vi "datalogging_sub.vi"(8 "Center Goal Position":i8, 9 "Path Selected":string, 10 "States Executed":T2[](array[typedef]), 11 "NXT/EV3 In":T1) -> (3 "NXT/EV3 Out":T1)   [LabVIEW 2012, in "Mecanum Drive.lvrbt"]
uses:
  Mecanum Drive.lvrbt
  State_Typ.ctl
  <vilib>/NXT/Subs/LVHSConnector.ctl
  <vilib>/NXT/LegoClasses/BrickReference/BrickReference.lvclass
  <vilib>/NXT/NXTIO Xnodes/NXTIONodeSubVIs/LEGOStopAllMotors.vi
  <vilib>/NXT/NXTIO Xnodes/NXTIONodeSubVIs/LEGOMoveAllMotors.vi
  <vilib>/NXT/NXTIO Xnodes/NXTIOXNode/NXTIO.xnode
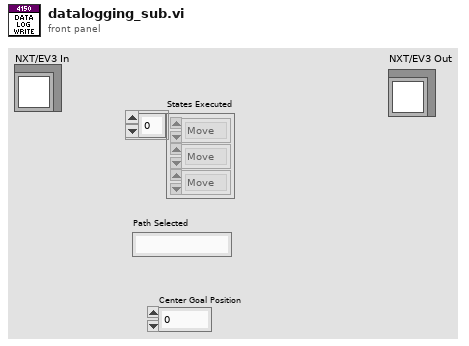
[diagram p1: front panel]
types:
  T1 = typedef "LVHSConnector.ctl" = refnum<class "BrickReference.lvclass">
  T2 = typedef "State_Typ.ctl" = enum16{"Move", "Check for Position 2", "Check for Position 3", "Stop"}
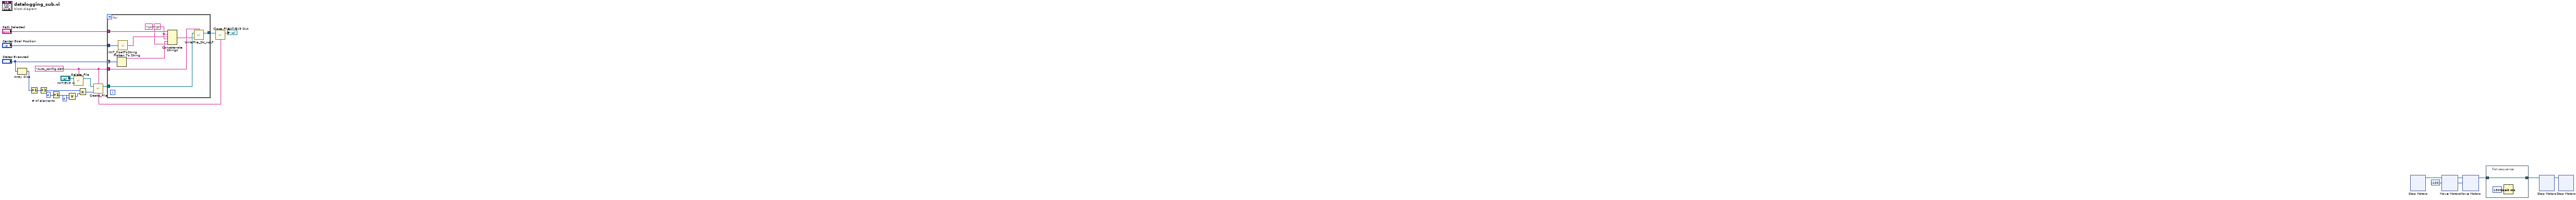
[diagram p0: block diagram]
diagram:
  w13 = 4  # # of elements
  w3 = "Auto_config.dat" ("Filename")
  w21 = i8 -100 ("Power/Speed 1")
  n1 = Array Size(array="States Executed") -> (size(s)=w6:i32)
  n2 = Increment(x=w6) -> (x+1=w14:i32)
  n3 = Increment(x=w14) -> (x+1=w9:i32)
  n4 = Increment(x=w13) -> (x+1=w12:i32)
  n5 = Multiply(x=w12, y=u32 4) -> (x*y=w11:u32)
  n6 = call <vilib>:"Delete_File.vi"("NXT/EV3"="NXT/EV3 In", "Filename"=w3) -> ("NXT/EV3"=w8:T1)  [unwired: 2 in]
  n7 = Multiply(x=w9, y=w11) -> (x*y=w15:u32)
  n8 = call <vilib>:"Create_File.vi"("File Size (256)"=w15, "NXT/EV3"=w8, "Filename"=w3) -> ("NXT/EV3"=w5:T1)  [unwired: 1 out]
  n9 = for {
    tunnel: "Path Selected" -> [w31]
    tunnel: "Center Goal Position" -> [w32]
    tunnel: "States Executed" -> [w26] mode=indexing
    tunnel: w5 -> [w34]
    tunnel: w3 -> [w24]
    tunnel: [w33] -> w4
    w29 = "\\t" ("string")
    n10 = Flatten To String(anything=w26) -> (data string=w25:string)  [unwired: 3 in, 2 out]
    n11 = call <vilib>:"NXT_floatToString.vi"("number"=w32) -> ("string"=w28:string)
    n12 = Concatenate Strings(w31, w29, w28, w29, w25, "\\n" ("string")) -> (w30:string)
    n13 = call <vilib>:"WriteFile_Str_noLF.vi"("String"=w30, "NXT/EV3"=w34, "Filename"=w24) -> ("NXT/EV3"=w33:T1)  [unwired: 1 in]
  }
  n14 = call <vilib>:"Close_File.vi"("NXT/EV3"=w4, "Filename"=w3) -> ("NXT/EV3"=→"NXT/EV3 Out":T1)  [unwired: 2 in]
  n15 = xnode "Stop Motors"() -> ("NXT/EV3"=w16:T1)  [unwired: 2 in]
  n16 = xnode "Move Motors"("Power/Speed 1"=w21, "NXT/EV3"=w16) -> ("NXT/EV3"=w20:T1)  [unwired: 1 in]
  n17 = xnode "Move Motors"("Power/Speed 1"=w21, "NXT/EV3"=w20) -> ("NXT/EV3"=w17:T1)  [unwired: 1 in]
  n18 = flat-sequence {
    tunnel: [w35] -> w19
    tunnel: w17 -> [w35]
    frame #0 {
      n19 = Wait (ms)(milliseconds to wait=u32 1500) -> ()  [unwired: 1 out]
    }
  }
  n20 = xnode "Stop Motors"("NXT/EV3"=w19) -> ("NXT/EV3"=w18:T1)  [unwired: 1 in]
  n21 = xnode "Stop Motors"("NXT/EV3"=w18) -> ()  [unwired: 1 in, 1 out]
